vi "minimum arguments.vi"() -> (3 "minimum arguments":i32)   [LabVIEW 2013]
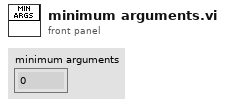
[diagram p1: front panel]
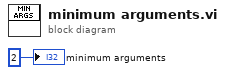
[diagram p0: block diagram]
diagram:
  "minimum arguments" <- 2 ("minimum arguments")
